vi "_UpdatePictureControl.vi"(6 "Zoom Factor":sgl=1.0, 8 "error in (no error)":errorcluster, 9 "Visible Frame":u32, 10 "Picture Control Reference":refnum<vi>, 11 "Center Object Reference":refnum<vi>) -> (0 "error out":errorcluster, 2 "New Picture":picture)   [LabVIEW 2017, in "CSM-Helper API with lvcsm Support.lvlib"]
uses:
  _csmHelper/API with lvcsm Support/CSM-Helper API with lvcsm Support.lvlib
  <vilib>/Utility/miscctls.llb/LVPointTypeDef.ctl
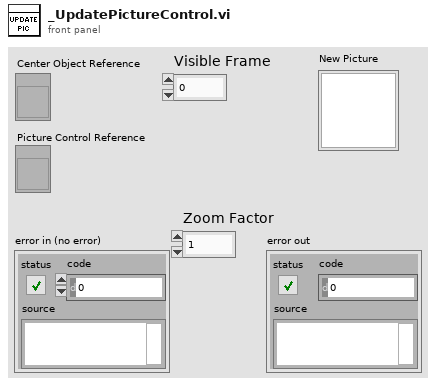
[diagram p1: front panel]
types:
  T1 = typedef "LVPointTypeDef.ctl" = cluster{"Horizontal":i16, "Vertical":i16}
  T2 = typedef "LVRectTypeDef.ctl" = cluster{"Left":i16, "Top":i16, "Right":i16, "Bottom":i16}
  T3 = typedef "LVBoundsTypeDef.ctl" = cluster{"Width":u32, "Height":u32}
  T4 = typedef "imagedata.ctl" = cluster{"image type":i32, "image depth":i32, "image":u8[], "mask":u8[], "colors":u32[], "Rectangle":cluster{"left":i16, "top":i16, "right":i16, "bottom":i16}}
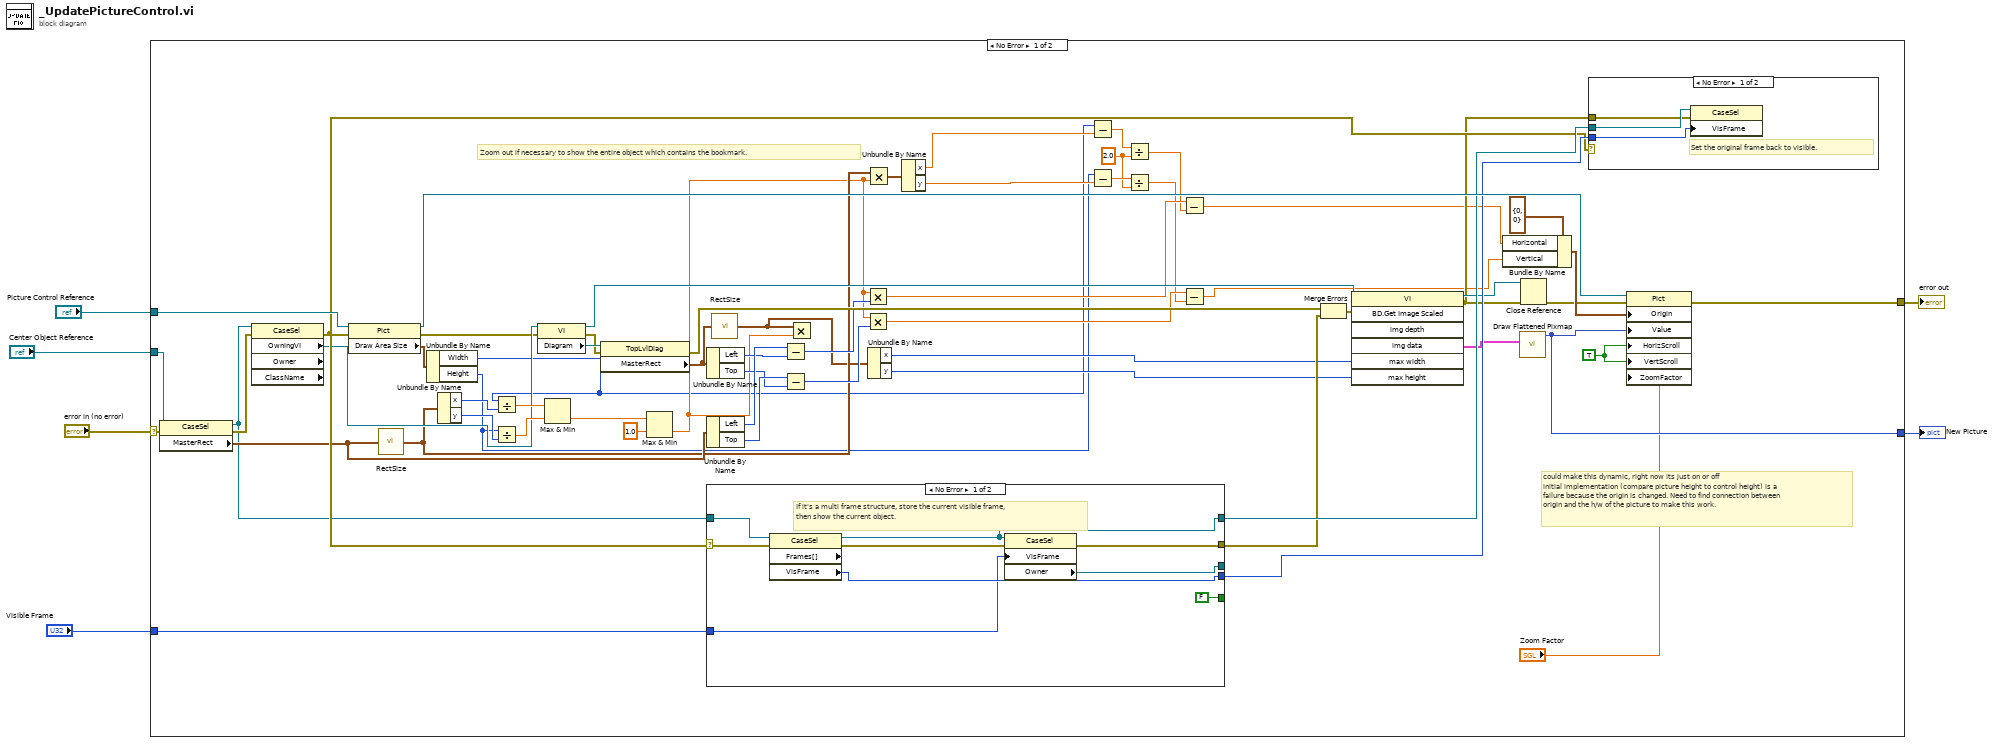
[diagram p0: block diagram]
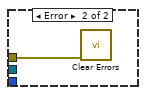
[diagram p2: hidden frame]
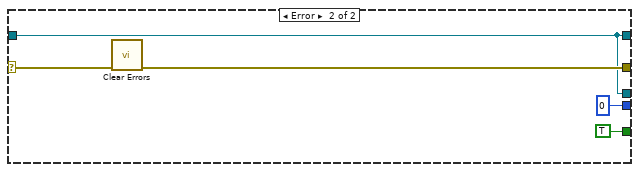
[diagram p3: hidden frame]
diagram:
  n1 = case shown="No Error" "error in (no error)" {
    selector: "error in (no error)" -> [w61 w87]
    tunnel: "Center Object Reference" -> [w65 _]
    tunnel: [w60 w87] -> w4
    tunnel: "Picture Control Reference" -> [w57 _]
    tunnel: "Visible Frame" -> [w9 _]
    tunnel: [w8 _] -> w1
    frame No Error {
      w11 = TRUE ("Vertical Scrollbar Visible")
      w24 = 2.0 ("y")
      # "could make this dynamic, right now its just on or off\ninitial implementation (compare picture height to control height) is a failure because the origin is changed. Need to find connection between origin and the h/w of the picture to make this work."
      # "Zoom out if necessary to show the entire object which contains the bookmark."
      n2 = property class="CaseSel"(reference=w65, error in=w61) -> (reference out=w10:refnum<vi>, error out=w62:errorcluster, "MasterRect"=w32:T2)
      n3 = property class="CaseSel" props=["OwningVI", "Owner", "ClassName"](reference=w10, error in=w62) -> (error out=w56:errorcluster, "OwningVI"=w50:refnum<vi>)  [unwired: 3 out]
      n4 = property class="Pict"(reference=w57, error in=w56) -> (reference out=w63:refnum<vi>, error out=w47:errorcluster, "Draw Area Size"=w51:T3)
      n5 = call <vilib>:"RectSize.vi"("rect"=w32) -> ("point"=w31:cluster{"x":i16, "y":i16})
      n6 = Unbundle By Name(w51) -> ("Width"=w14:u32, "Height"=w13:u32)
      n7 = Unbundle By Name(w31) -> ("x"=w55:i16, "y"=w54:i16)
      n8 = Divide(x=w14, y=w55) -> (x/y=w53:dbl)
      n9 = Divide(x=w13, y=w54) -> (x/y=w52:dbl)
      n10 = property class="VI"(reference=w50, error in=w47) -> (reference out=w49:refnum<vi>, error out=w64:errorcluster, "Diagram"=w68:refnum<vi>)
      n11 = Max & Min(x=w53, y=w52) -> (min(x,y)=w41:dbl)  [unwired: 1 out]
      n12 = property class="TopLvlDiag"(reference=w68, error in=w64) -> (error out=w46:errorcluster, "MasterRect"=w33:T2)  [unwired: 1 out]
      n13 = Max & Min(x=w41, y=1.0) -> (min(x,y)=w30:dbl)  [unwired: 1 out]
      n14 = Unbundle By Name(w33) -> ("Left"=w38:i16, "Top"=w35:i16)
      n15 = Unbundle By Name(w32) -> ("Left"=w39:i16, "Top"=w37:i16)
      n16 = case shown="No Error" w56 {
        selector: w56 -> [w78 w86]
        tunnel: w10 -> [w81 w82]
        tunnel: [w76 w85] -> w45
        tunnel: [w80 u32 0 ("VisFrame")] -> w59
        tunnel: [w79 w82] -> w58
        tunnel: [FALSE TRUE] -> _
        tunnel: [w74 w82] -> _
        tunnel: w9 -> [w73 _]
        frame No Error {
          # "If it's a multi frame structure, store the current visible frame,\nthen show the current object."
          n17 = property class="CaseSel" props=["Frames[]", "VisFrame"](reference=w81, error in=w78) -> (reference out=w79:refnum<vi>, error out=w77:errorcluster, "VisFrame"=w80:u32)  [unwired: 1 out]
          n18 = property class="CaseSel"(reference=w79, error in=w77, "VisFrame"=w73) -> (error out=w76:errorcluster, "Owner"=w74:refnum<vi>)  [unwired: 1 out]
        }
        frame Error {
          n19 = call <vilib>:"Clear Errors.vi"("error in (no error)"=w86) -> ("error out"=w85:errorcluster)  [unwired: 5 in, 1 out]
        }
      }
      n20 = call <vilib>:"RectSize.vi"("rect"=w33) -> ("point"=w12:cluster{"x":i16, "y":i16})
      n21 = Subtract(x=w39, y=w38) -> (x-y=w36:i16)
      n22 = Subtract(x=w37, y=w35) -> (x-y=w34:i16)
      n23 = Multiply(x=w12, y=w30) -> ()  [unwired: 1 out]
      n24 = Multiply(x=w30, y=w36) -> (x*y=w23:dbl)
      n25 = Multiply(x=w30, y=w34) -> (x*y=w20:dbl)
      n26 = Multiply(x=w31, y=w30) -> (x*y=w29:cluster{"x":dbl, "y":dbl})
      n27 = Unbundle By Name(w12) -> ("x"=w16:i16, "y"=w15:i16)
      n28 = Unbundle By Name(w29) -> ("x"=w28:dbl, "y"=w26:dbl)
      n29 = Subtract(x=w14, y=w28) -> (x-y=w27:dbl)
      n30 = Subtract(x=w13, y=w26) -> (x-y=w25:dbl)
      n31 = Divide(x=w27, y=w24) -> (x/y=w22:dbl)
      n32 = Divide(x=w25, y=w24) -> (x/y=w19:dbl)
      n33 = Subtract(x=w23, y=w22) -> (x-y=w21:dbl)
      n34 = Subtract(x=w20, y=w19) -> (x-y=w18:dbl)
      n35 = Merge Errors(w46, w45) -> (w44:errorcluster)
      n36 = invoke class="VI" method="BD.Get Image Scaled"(reference=w49, error in=w44, "max width"=w16, "max height"=w15) -> (reference out=w48:refnum<vi>, error out=w43:errorcluster, "img data"=w17:T4)  [unwired: 3 in, 4 out]
      n37 = Bundle By Name(cluster=T1 {"Horizontal"=0, "Vertical"=0} ("Origin"), "Horizontal"=w21, "Vertical"=w18) -> (w66:T1)
      n38 = call <vilib>:"Draw Flattened Pixmap.vi"("image data"=w17) -> ("new picture"=w8:picture)  [unwired: 8 in]
      n39 = Close Reference(reference=w48, error in (no error)=w43) -> (error out=w42:errorcluster)
      n40 = case shown="No Error" w56 {
        tunnel: w59 -> [w71 _]
        tunnel: w58 -> [w70 _]
        tunnel: w43 -> [w69 w72]
        frame No Error {
          # "Set the original frame back to visible."
          n41 = property class="CaseSel"(reference=w70, error in=w69, "VisFrame"=w71) -> ()  [unwired: 2 out]
        }
        frame Error {
          n42 = call <vilib>:"Clear Errors.vi"("error in (no error)"=w72) -> ()  [unwired: 5 in, 2 out]
        }
      }
      n43 = property on="Property Node" class="Pict"(reference=w63, error in=w42, "Origin"=w66, "Value"=w8, "HorizScroll"=w11, "VertScroll"=w11, "ZoomFactor"="Zoom Factor") -> (error out=w60:errorcluster)  [unwired: 1 out]
    }
    frame Error {
    }
  }
  "error out" <- w4
  "New Picture" <- w1
